vi "Varint Decoder.vi"   [LabVIEW 2017]
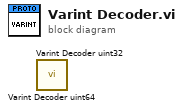
[diagram p0: block diagram]
diagram:
  n1 = call "Varint Decoder uint64.vi"() -> ()  [unwired: 8 in, 4 out]
  n2 = call "Varint Decoder uint32.vi"() -> ()  [unwired: 8 in, 4 out]
